vi "PH_Beamline.get i attribute.vi"(0 "i ref in":refnum<vi>, 5 "error in (no error)":errorcluster) -> (14 "i ref out":refnum<vi>, 16 "i attribute":T1={"GUI Refs"={"PA ok"=refnum, "MA ok"=refnum, "fs FE ok"=refnum, "ns FE ok"=refnum, "PA ED ok"=refnum, "MAS ok"=refnum, "Booster ok"=refnum, "Mirrortower ok"=refnum, "In.-Box ok"=refnum, "Compressor ok"=refnum, "Experiment LB ok"=refnum, "Experiment LL ok"=refnum, "PHELIX_Beckhoff_Watchdog"=refnum, "Shutters closed"=refnum, "uOPA ok"=refnum, "Vacuum no shotcond Comp LB"=refnum}, "Refs BL MA"=[], "Refs BL MA-IB"=[], "Refs BL fs"=[], "Refs BL PA ED"=[], "Refs BL MAS"=[], "Refs BL Boo"=[], "Refs BL ns"=[], "Refs BL Mirrortower"=[], "Refs BL Compressor"=[], "Refs BL Exp LB"=[], "Radiation Safety"={"Exp Laserbay"={"Ref Op Mode"=refnum, "Ref Laserbay evacuated"=refnum, "Tagname LB evacuated"="N/A", "Shot Mode"=0, "Laserbay evacuated?"=0, "Tagname HV room locked"="N/A", "HV room locked?"=0, "Ref HV room locked"=refnum, "Tagname bridged?"="N/A", "Ref Bridge"=refnum, "I<1E18W/cm²"=FALSE}, "Exp Laserlab"={"Ref Op Mode"=refnum, "Ref Laserlab evacuated"=refnum, "Tagname LL evacuated"="N/A", "Shot Mode"=0, "Laserlab evacuated?"=0, "Tagname bridged?"="N/A", "Ref Bridge"=refnum, "I<1E18W/cm²"=FALSE}}, "Refs BL LL"=[], "PP Igni Heating GUI Refs"=[], "PP Igni Heating Tagnames "=[], "Refs BL PA"={"undelayed Line before Shutter"=[], "undelayed Line after Shutter"=[], "before Bypass"=[], "delayed Line before Shutter"=[], "delayed Line after Shutter"=[], "before Shutter Input"=[], "after Shutter Input"=[], "Bypass"=[], "before Shutter Exit"=[], "after Shutter Exit"=[], "to MA"=[], "to Lab"=[]}, "BL"={"YLF_BL_Status"=-1, "fs_BL_Status"=-1, "fs_YLF_BL_Status"=-1, "ns_BL_Status"=-1, "PA_Input_BL_Status"=-1, "PA_UnDelay_BL_Status"=-1, "PA_Delay_BL_Status"=-1, "PA_BL_Status"=-1, "PA_Bypass_BL_Status"=-1, "PA_Exit_BL_Status"=-1, "PA_LL_BL_Status"=-1, "LL_BL_Status"=-1, "PA_MA_BL_Status"=-1, "MA_Exit_BL_Status"=-1, "MA_Z6_BL_Status"=-1, "Z6_BL_Status"=-1, "MA_LB_BL_Status"=-1, "LB_TB2_BL_Status"=-1, "PA_before_Bypass_BL_Status"=-1, "LB_TB3_BL_Status"=-1}, "State Subsystems"={"PA"=FALSE, "MA"=FALSE, "ns FE"=FALSE, "fs FE"=FALSE, "PA ED"=FALSE, "In.-Box"=FALSE, "MAS"=FALSE, "Booster"=FALSE, "Mirrortower"=FALSE, "Compressor"=FALSE, "Experiment LB"=FALSE, "Experiment LL"=FALSE, "uOPA"=FALSE}, "Status Subscriber Information"={"fs Swich YLF"={"Index of element"=-1, "Attributeset"=enum."Boolean Status Service Subscriber"}, "fs Exit Shutter"={"Index of element"=-1, "Attributeset"=enum."Boolean Status Service Subscriber"}, "ns Exit Shutter"={"Index of element"=-1, "Attributeset"=enum."Boolean Status Service Subscriber"}, "PA Input Shutter"={"Index of element"=-1, "Attributeset"=enum."Boolean Status Service Subscriber"}, "PA PC WP"={"Index of element"=-1, "Attributeset"=enum."Boolean Status Service Subscriber"}, "PA PC WP 2"={"Index of element"=-1, "Attributeset"=enum."Boolean Status Service Subscriber"}, "PA Bypass In"={"Index of element"=-1, "Attributeset"=enum."Boolean Status Service Subscriber"}, "PA Bypass Out"={"Index of element"=-1, "Attributeset"=enum."Boolean Status Service Subscriber"}, "PA CH 1"={"Index of element"=-1, "Attributeset"=enum."Boolean Status Service Subscriber"}, "PA delayed"={"Index of element"=-1, "Attributeset"=enum."Boolean Status Service Subscriber"}, "PA non delayed"={"Index of element"=-1, "Attributeset"=enum."Boolean Status Service Subscriber"}, "PA Exit Shutter"={"Index of element"=-1, "Attributeset"=enum."Boolean Status Service Subscriber"}, "PA Switch Lab"={"Index of element"=-1, "Attributeset"=enum."Boolean Status Service Subscriber"}, "PA Bridge CH Input MA"={"Index of element"=-1, "Attributeset"=enum."Boolean Status Service Subscriber"}, "MA Diffusor IB"={"Index of element"=-1, "Attributeset"=enum."Boolean Status Service Subscriber"}, "MA IB Ready"={"Index of element"=-1, "Attributeset"=enum."Boolean Status Service Subscriber"}, "MA CH 1"={"Index of element"=-1, "Attributeset"=enum."Boolean Status Service Subscriber"}, "MA CH 2"={"Index of element"=-1, "Attributeset"=enum."Boolean Status Service Subscriber"}, "MA CH 3"={"Index of element"=-1, "Attributeset"=enum."Boolean Status Service Subscriber"}, "MA CH 4"={"Index of element"=-1, "Attributeset"=enum."Boolean Status Service Subscriber"}, "MA Shutter Align Cam"={"Index of element"=-1, "Attributeset"=enum."Boolean Status Service Subscriber"}, "MA Position MM5"={"Index of element"=-1, "Attributeset"=enum."Boolean Status Service Subscriber"}, "Calorimeter Switch"={"Index of element"=-1, "Attributeset"=enum."Boolean Status Service Subscriber"}, "BL Z6 CH 9"={"Index of element"=-1, "Attributeset"=enum."Boolean Status Service Subscriber"}, "BL Z6 Beamdump"={"Index of element"=-1, "Attributeset"=enum."Boolean Status Service Subscriber"}, "BL Z6 Shutter"={"Index of element"=-1, "Attributeset"=enum."Boolean Status Service Subscriber"}, "COS Sensitivity Switch"={"Index of element"=-1, "Attributeset"=enum."Boolean Status Service Subscriber"}, "Exp LB Shutter"={"Index of element"=-1, "Attributeset"=enum."Boolean Status Service Subscriber"}, "Exp LB TB 2"={"Index of element"=-1, "Attributeset"=enum."Boolean Status Service Subscriber"}, "Exp LB TB 3"={"Index of element"=-1, "Attributeset"=enum."Boolean Status Service Subscriber"}, "PA LL Input CH"={"Index of element"=-1, "Attributeset"=enum."Boolean Status Service Subscriber"}, "PA LL Output CH"={"Index of element"=-1, "Attributeset"=enum."Boolean Status Service Subscriber"}, "LL Comp Input Shutter"={"Index of element"=-1, "Attributeset"=enum."Boolean Status Service Subscriber"}, "LL Comp Output Shutter"={"Index of element"=-1, "Attributeset"=enum."Boolean Status Service Subscriber"}, "LL Comp FF Shutter"={"Index of element"=-1, "Attributeset"=enum."Boolean Status Service Subscriber"}, "Exp LL Shutter"={"Index of element"=0, "Attributeset"=enum."Boolean Status Service Subscriber"}, "MA IM In IB"={"Index of element"=0, "Attributeset"=enum."Boolean Status Service Subscriber"}, "MA IM Out IB"={"Index of element"=0, "Attributeset"=enum."Boolean Status Service Subscriber"}, "MA DB In IB"={"Index of element"=0, "Attributeset"=enum."Boolean Status Service Subscriber"}, "MA DB Out IB"={"Index of element"=0, "Attributeset"=enum."Boolean Status Service Subscriber"}, "Exp LB Shutter Interlock"={"Index of element"=0, "Attributeset"=enum."Boolean Status Service Subscriber"}, "Exp LL Shutter Interlock"={"Index of element"=0, "Attributeset"=enum."Boolean Status Service Subscriber"}, "MM1 Force Sensor"={"Index of element"=0, "Attributeset"=enum."Boolean Status Service Subscriber"}}, "Refs BL uOPA"=[], "PA_Input_2_Beam_6PWpGUI not linked?"=FALSE, "PA_Input_Delay_6PGUI not linked?"=FALSE, "Settings"={"PA Doublepass Mode"=FALSE, "Compressor Vaccuum LB not relevant"=FALSE, "Windowshutter TB2 not relevant"=FALSE, "Windowshutter TB3 not relevant"=FALSE}} {"Radiation Safety"."Exp Laserlab"."Laserlab evacuated?" items=["no info", "LL not evacuated", "LL evacuated"]; "Radiation Safety"."Exp Laserlab"."Shot Mode" items=["no info", "no Shotmode", "Shotmode"]; "Radiation Safety"."Exp Laserbay"."HV room locked?" items=["no info", "HV room open", "HV room locked"]; "Radiation Safety"."Exp Laserbay"."Laserbay evacuated?" items=["no info", "LB not evacuated", "LB evacuated"]; "Radiation Safety"."Exp Laserbay"."Shot Mode" items=["no info", "no Shotmode", "Shotmode"]}, 19 "error out":errorcluster)   [LabVIEW 2014, in "PH_Beamline.lvlib"]
doc: "Gets the i attribute data of an object.\n\nLicense Agreement for this software:\n\nCopyright (C)\nGesellschaft für Schwerionenforschung, GSI\nPlanckstr. 1\n64291 Darmstadt\nGermany\n\nContact: D.Beck@gsi.de \n\nThis program is free software; you can redistribute it and/or modify it under the terms of the GNU General Public License as published by the Free Software Foundation; either version 2 of the license, or (at your option) any later version.\n\nThis program is distributed in the hope that it will be useful, but WITHOUT ANY WARRANTY; without even the implied warranty of MERCHANTABILITY or FITNESS FOR A PARTICULAR PURPOSE. See the GNU General License for more details (http://www.gnu.org).\n\nGesellschaft für Schwerionenforschung, GSI\nPlanckstr. 1, 64291 Darmstadt, Germany\nFor all questions and ideas contact: M.Richter@gsi.de, H.Brand@gsi.de or D.Beck@gsi.de.\nLast update: 17-JUN-2004"
uses:
  PH_Beamline.lvlib
  PH_Beamline.i attribute.ctl
  PH_Beamline.Operation Mode.ctl
  PH_Beamline.Status Subscriber Information.ctl
  PH_BL-Master/PH_BL-Master.Status Subscriber Information.ctl
  PH_BL-Master/PH_BL-Master.Attribute Set.ctl
  PH_Beamline_Chief/PH_Beamline_Chief.Settings.ctl
  PH_BL-Master/PH_BL-Master.lvlib
  PH_Beamline_Chief/PH_Beamline_Chief.lvlib
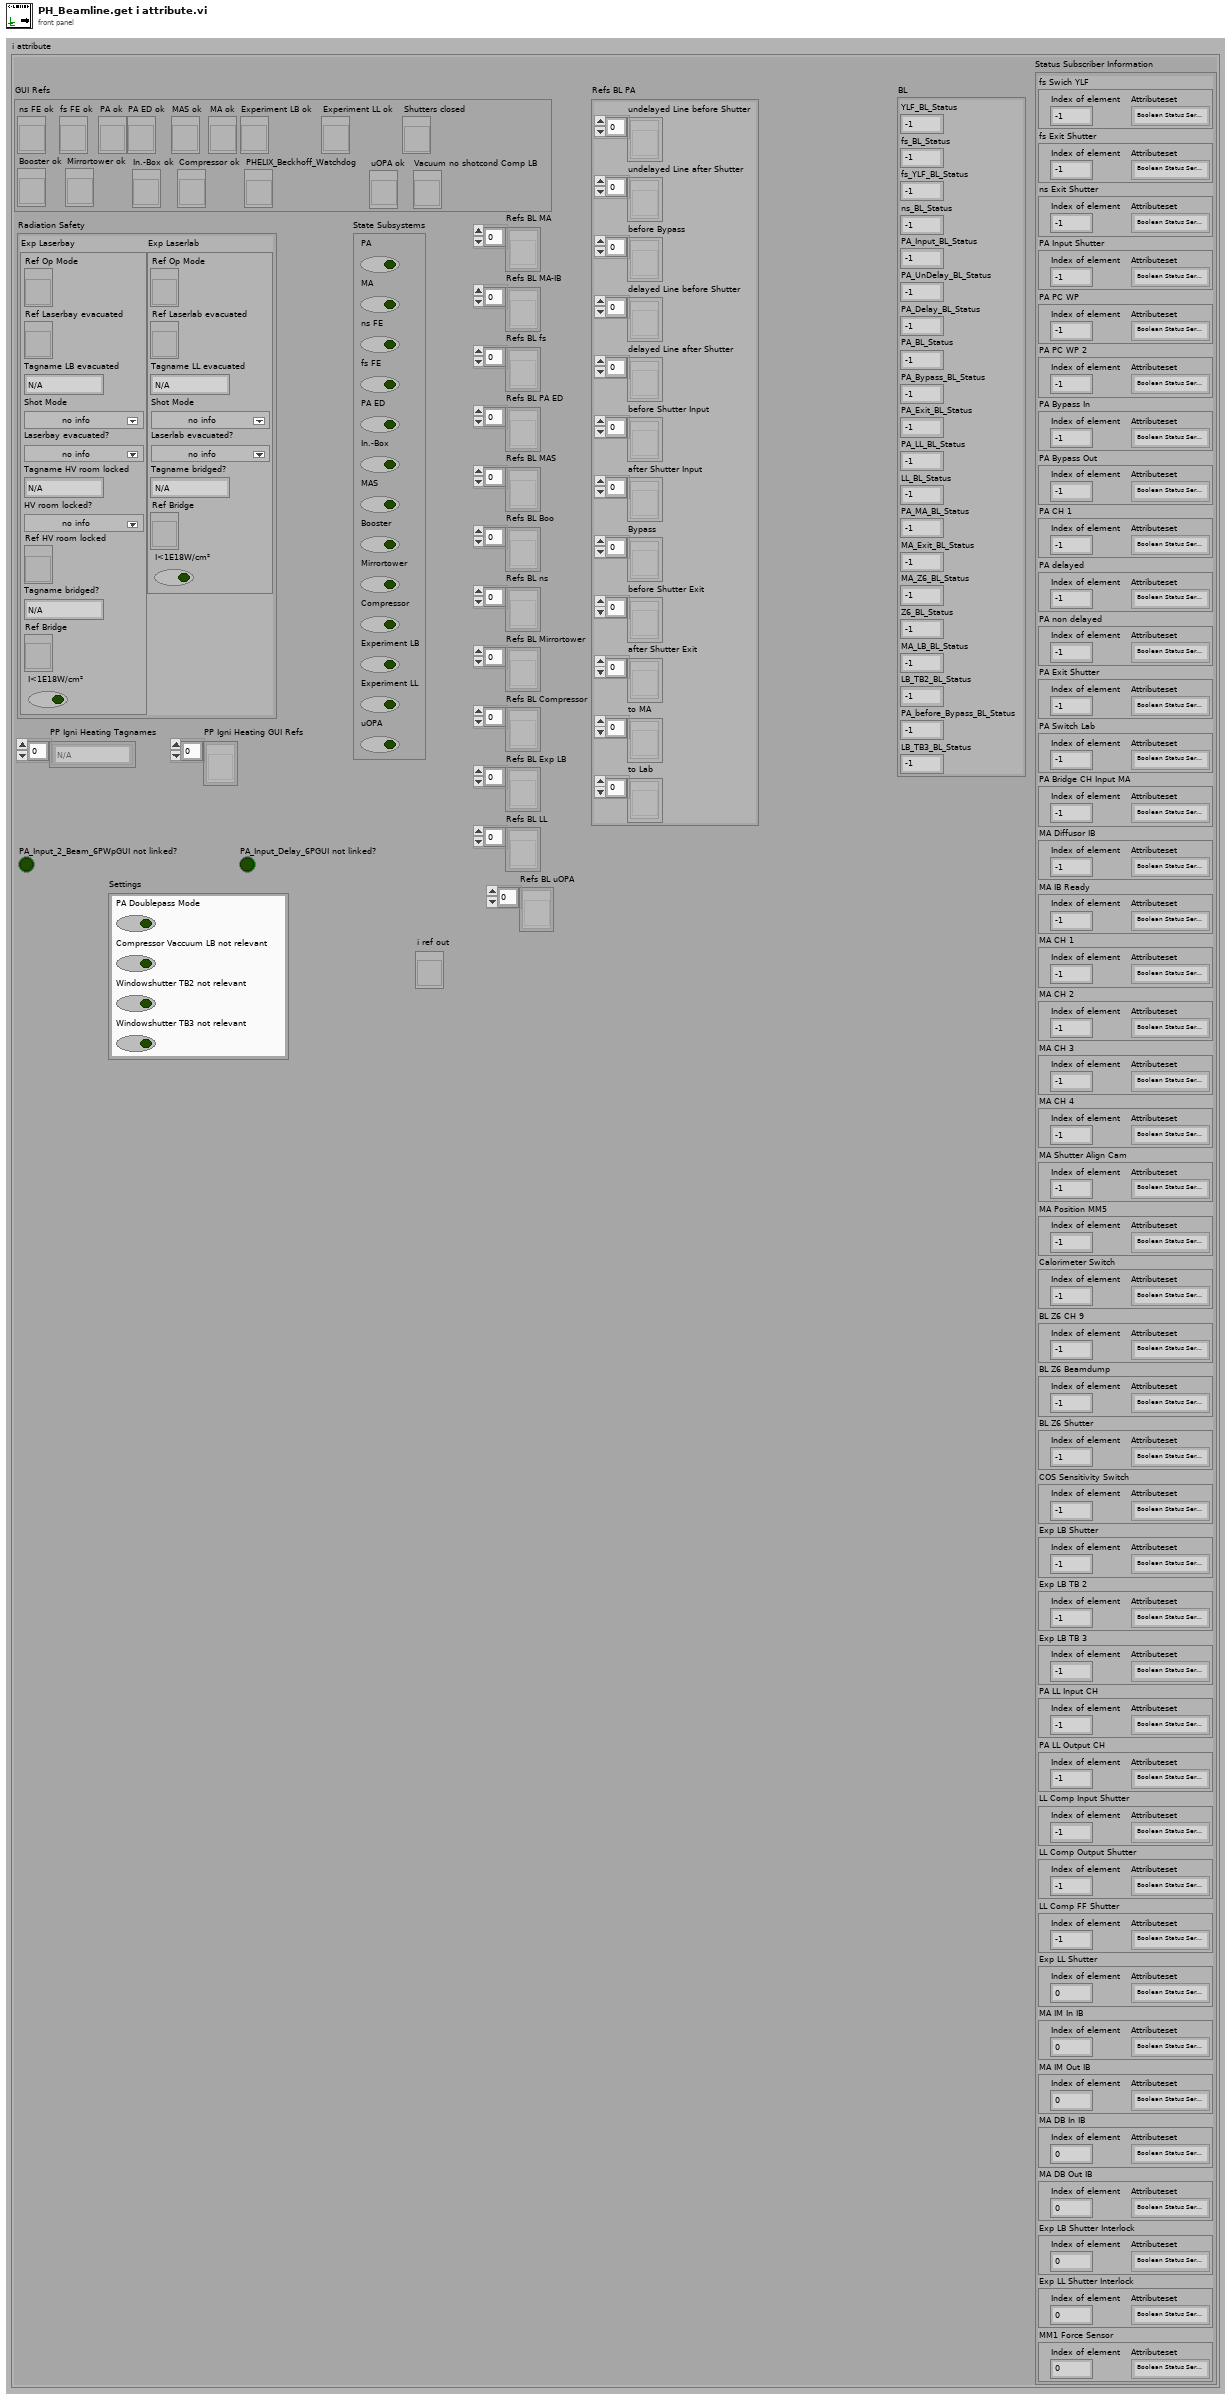
[diagram p1: front panel]
types:
  T1 = typedef "PH_Beamline.lvlib/PH_Beamline.i attribute.ctl" = cluster{"GUI Refs":cluster{"PA ok":refnum<vi>, "MA ok":refnum<vi>, "fs FE ok":refnum<vi>, "ns FE ok":refnum<vi>, "PA ED ok":refnum<vi>, "MAS ok":refnum<vi>, "Booster ok":refnum<vi>, "Mirrortower ok":refnum<vi>, "In.-Box ok":refnum<vi>, "Compressor ok":refnum<vi>, "Experiment LB ok":refnum<vi>, "Experiment LL ok":refnum<vi>, "PHELIX_Beckhoff_Watchdog":refnum<vi>, "Shutters closed":refnum<vi>, "uOPA ok":refnum<vi>, "Vacuum no shotcond Comp LB":refnum<vi>}, "Refs BL MA":refnum<vi>[], "Refs BL MA-IB":refnum<vi>[], "Refs BL fs":refnum<vi>[], "Refs BL PA ED":refnum<vi>[], "Refs BL MAS":refnum<vi>[], "Refs BL Boo":refnum<vi>[], "Refs BL ns":refnum<vi>[], "Refs BL Mirrortower":refnum<vi>[], "Refs BL Compressor":refnum<vi>[], "Refs BL Exp LB":refnum<vi>[], "Radiation Safety":cluster{"Exp Laserbay":cluster{"Ref Op Mode":refnum<vi>, "Ref Laserbay evacuated":refnum<vi>, "Tagname LB evacuated":string, "Shot Mode":T2, "Laserbay evacuated?":i32, "Tagname HV room locked":string, "HV room locked?":i32, "Ref HV room locked":refnum<vi>, "Tagname bridged?":string, "Ref Bridge":refnum<vi>, "I<1E18W/cm²":bool}, "Exp Laserlab":cluster{"Ref Op Mode":refnum<vi>, "Ref Laserlab evacuated":refnum<vi>, "Tagname LL evacuated":string, "Shot Mode":T2, "Laserlab evacuated?":i32, "Tagname bridged?":string, "Ref Bridge":refnum<vi>, "I<1E18W/cm²":bool}}, "Refs BL LL":refnum<vi>[], "PP Igni Heating GUI Refs":refnum<vi>[], "PP Igni Heating Tagnames ":string[], "Refs BL PA":cluster{"undelayed Line before Shutter":refnum<vi>[], "undelayed Line after Shutter":refnum<vi>[], "before Bypass":refnum<vi>[], "delayed Line before Shutter":refnum<vi>[], "delayed Line after Shutter":refnum<vi>[], "before Shutter Input":refnum<vi>[], "after Shutter Input":refnum<vi>[], "Bypass":refnum<vi>[], "before Shutter Exit":refnum<vi>[], "after Shutter Exit":refnum<vi>[], "to MA":refnum<vi>[], "to Lab":refnum<vi>[]}, "BL":cluster{"YLF_BL_Status":i32, "fs_BL_Status":i32, "fs_YLF_BL_Status":i32, "ns_BL_Status":i32, "PA_Input_BL_Status":i32, "PA_UnDelay_BL_Status":i32, "PA_Delay_BL_Status":i32, "PA_BL_Status":i32, "PA_Bypass_BL_Status":i32, "PA_Exit_BL_Status":i32, "PA_LL_BL_Status":i32, "LL_BL_Status":i32, "PA_MA_BL_Status":i32, "MA_Exit_BL_Status":i32, "MA_Z6_BL_Status":i32, "Z6_BL_Status":i32, "MA_LB_BL_Status":i32, "LB_TB2_BL_Status":i32, "PA_before_Bypass_BL_Status":i32, "LB_TB3_BL_Status":i32}, "State Subsystems":cluster{"PA":bool, "MA":bool, "ns FE":bool, "fs FE":bool, "PA ED":bool, "In.-Box":bool, "MAS":bool, "Booster":bool, "Mirrortower":bool, "Compressor":bool, "Experiment LB":bool, "Experiment LL":bool, "uOPA":bool}, "Status Subscriber Information":T3, "Refs BL uOPA":refnum<vi>[], "PA_Input_2_Beam_6PWpGUI not linked?":bool, "PA_Input_Delay_6PGUI not linked?":bool, "Settings":T6}
  T2 = typedef "PH_Beamline.lvlib/PH_Beamline.Operation Mode.ctl" = i32
  T3 = typedef "PH_Beamline.lvlib/PH_Beamline.Status Subscriber Information.ctl" = cluster{"fs Swich YLF":T4, "fs Exit Shutter":T4, "ns Exit Shutter":T4, "PA Input Shutter":T4, "PA PC WP":T4, "PA PC WP 2":T4, "PA Bypass In":T4, "PA Bypass Out":T4, "PA CH 1":T4, "PA delayed":T4, "PA non delayed":T4, "PA Exit Shutter":T4, "PA Switch Lab":T4, "PA Bridge CH Input MA":T4, "MA Diffusor IB":T4, "MA IB Ready":T4, "MA CH 1":T4, "MA CH 2":T4, "MA CH 3":T4, "MA CH 4":T4, "MA Shutter Align Cam":T4, "MA Position MM5":T4, "Calorimeter Switch":T4, "BL Z6 CH 9":T4, "BL Z6 Beamdump":T4, "BL Z6 Shutter":T4, "COS Sensitivity Switch":T4, "Exp LB Shutter":T4, "Exp LB TB 2":T4, "Exp LB TB 3":T4, "PA LL Input CH":T4, "PA LL Output CH":T4, "LL Comp Input Shutter":T4, "LL Comp Output Shutter":T4, "LL Comp FF Shutter":T4, "Exp LL Shutter":T4, "MA IM In IB":T4, "MA IM Out IB":T4, "MA DB In IB":T4, "MA DB Out IB":T4, "Exp LB Shutter Interlock":T4, "Exp LL Shutter Interlock":T4, "MM1 Force Sensor":T4}
  T4 = typedef "PH_BL-Master.lvlib/PH_BL-Master.Status Subscriber Information.ctl" = cluster{"Index of element":i32, "Attributeset":T5}
  T5 = typedef "PH_BL-Master.lvlib/PH_BL-Master.Attribute Set.ctl" = enum16{"Boolean Status Service Subscriber", "Picture Status Service Subscriber"}
  T6 = typedef "PH_Beamline_Chief.lvlib/PH_Beamline_Chief.Settings.ctl" = cluster{"PA Doublepass Mode":bool, "Compressor Vaccuum LB not relevant":bool, "Windowshutter TB2 not relevant":bool, "Windowshutter TB3 not relevant":bool}
  T7 = enum16{"SetAttribute", "GetAttribute", "CreateAttribute", "DestroyAttribute", "DestroyAllAtributes"}
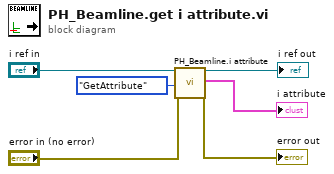
[diagram p0: block diagram]
diagram:
  n1 = call "PH_Beamline.i attribute.vi"("VI Refnum"="i ref in", "Action"=T7."GetAttribute", "error in (no error)"="error in (no error)") -> ("VI Refnum out"=→"i ref out":refnum<vi>, "CLASS.i attribute out"=→"i attribute":T1, "error out"=→"error out":errorcluster)  [unwired: 14 in]
